vi "State2-Parallel.vi"(9 "Numeric 7":dbl, 11 "Numeric in":dbl) -> (1 "Init Left/Right Speed 3":u32, 2 "Left/Right":enum16{"Left", "Right", "Stop"}(ring), 3 "Front/Back 2":enum16{"Forward", "Backward", "Stop"}(ring), 4 "Cluster":T2, 5 "Enum":T1)   [LabVIEW 2014]
uses:
  FPGA Bitfiles/Parking States Indicators.ctl
  FPGA Bitfiles/Parking States.ctl
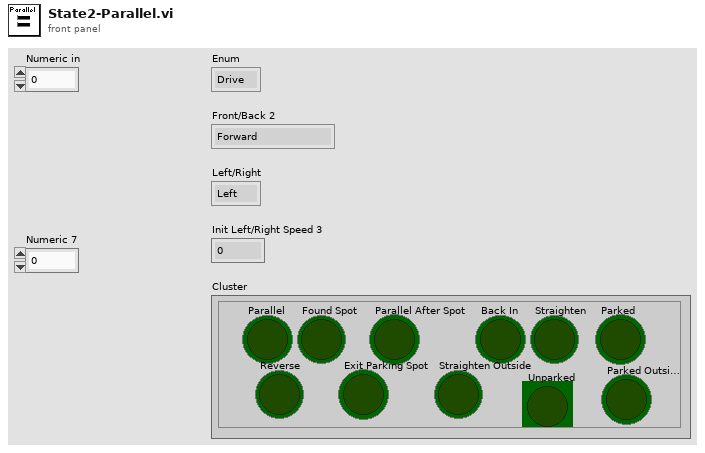
[diagram p1: front panel]
types:
  T1 = typedef "Parking States.ctl" = enum16{"Drive", "Parallel", "Found Spot", "Parallel After Spot", "Back In", "Straighten", "Parked", "Reverse", "Exit Parking Spot", "Straighten Outside", "Unparked", "Parked Outside"}
  T2 = typedef "Parking States Indicators.ctl" = cluster{"Parallel":bool, "Found Spot":bool, "Parallel After Spot":bool, "Back In":bool, "Straighten":bool, "Parked":bool, "Reverse":bool, "Exit Parking Spot":bool, "Straighten Outside":bool, "Unparked":bool, "Parked Outside":bool}
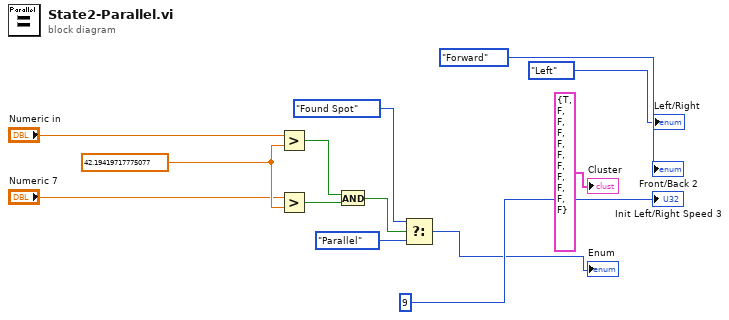
[diagram p0: block diagram]
diagram:
  w8 = 42.19419717775077 ("Distance to detect parking spot")
  n1 = Greater?(x="Numeric in", y=w8) -> (0:w1:bool)
  n2 = Greater?(x="Numeric 7", y=w8) -> (0:w2:bool)
  n3 = And(x=w1, y=w2) -> (x .and. y?=w3:bool)
  n4 = Select(t=Parking_States."Found Spot", s=w3, f=Parking_States."Parallel") -> (s? t:f=→"Enum":T1)
  "Init Left/Right Speed 3" <- u32 9 ("Init Left/Right Speed in")
  "Cluster" <- T2 {"Parallel"=TRUE, "Found Spot"=FALSE, "Parallel After Spot"=FALSE, "Back In"=FALSE, "Straighten"=FALSE, "Parked"=FALSE, "Reverse"=FALSE, "Exit Parking Spot"=FALSE, "Straighten Outside"=FALSE, "Unparked"=FALSE, "Parked Outside"=FALSE} ("Cluster")
  "Front/Back 2" <- enum16{"Forward", "Backward", "Stop"}."Forward" ("Front/Back 2")
  "Left/Right" <- enum16{"Left", "Right", "Stop"}."Left" ("Left/Right")
